vi "Main.vi"() -> ()   [LabVIEW 2013]
uses:
  <vilib>/Platform/TimedLoop/XDataNode/timing_clust.ctl
  <vilib>/Platform/TimedLoop/XDataNode/nitl_modes.ctl
  <vilib>/Platform/TimedLoop/XDataNode/wakeup.ctl
  <vilib>/Utility/file.llb/Write To Spreadsheet File (DBL).vi
  <vilib>/platform/TimedLoop/XDataNode/XDataNode.xnode
  <vilib>/Platform/TimedLoop/XDataNode/XDNodeRunTimeDep.lvlib
panel:
  out "X-axis acceleration [g]":dbl(knob) scale=-2.0..2.0
  out "Acquired data":cluster{dbl[], dbl[]}(graph)
  in  "[ESC]":bool
  in  "logfile base name":string="logfile"
  out "logfile name":path
  out "USB flash drive info":string
  out "folder names":string[](array[string])
  out "filenames":string[](array[string])
  # "USB Flash Drive demo"
  # "1. Insert USB flash drive\n2. Enter logfile base name\n3. Run the VI\n4. Move NI myRIO to see onboard\n    accelerometer activity\n5. Stop the VI to save\n    acquired acceleration data to\n    logfile on USB flash drive"
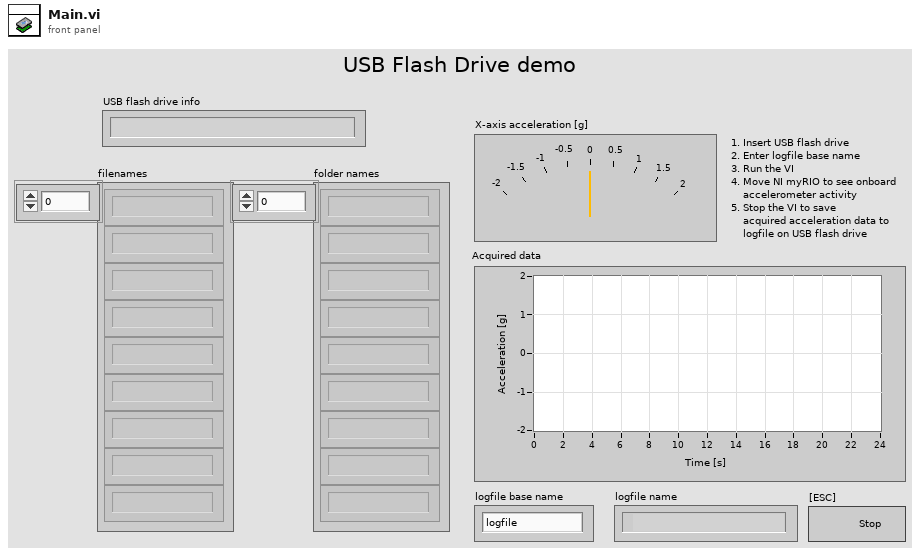
[diagram p1: front panel]
types:
  T1 = typedef "XDNodeRunTimeDep.lvlib/timing_clust.ctl" = cluster{"Expected End [f-1]":u64, "Actual End [f-1]":u64, "Finished Late? [f-1]":bool, "Expected End [i-1]":u64, "Actual End [i-1]":u64, "Finished Late? [i-1]":bool, "Expected Start [i]":u64, "Actual Start [i]":u64, "Expected Start [f]":u64, "Actual Start [f]":u64, "Source Name":string, "Structure Name":string, "Period":i64, "Deadline":i64, "Offset":i64, "Start":i64, "Priority":i32, "Timeout":i32, "Mode":T2, "Wakeup Reason":T3, "Error":errorcluster, "Source Type":string, "Secondary Source Type":string, "Global End Time":u64, "Global Start Time":u64, "Frame Duration":u64, "Iteration Duration":u64, "Assigned CPU":i32, "I/O Scan Engine Mode":u32}
  T2 = typedef "XDNodeRunTimeDep.lvlib/nitl_modes.ctl" = enum32{"No Change", "Process missed periods, maintain original phase", "Discard missed periods, maintain original phase", "Process missed periods, ignore original phase", "Discard missed periods, ignore original phase"}
  T3 = typedef "XDNodeRunTimeDep.lvlib/wakeup.ctl" = enum32{"Normal", "Aborted", "Asynchronous wakeup", "Timing source error", "Timed loop error", "Timeout"}
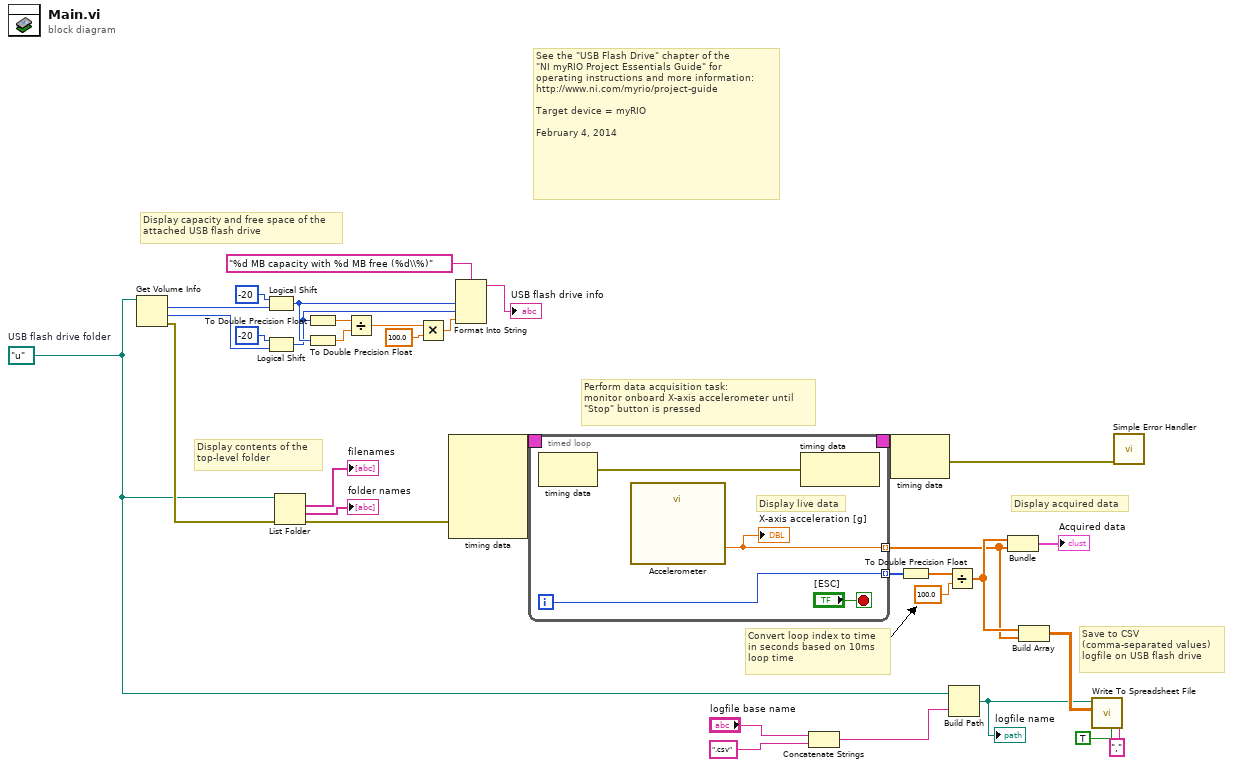
[diagram p0: block diagram]
diagram:
  w1 = path "u:/"  # USB flash drive folder
  # "See the \"USB Flash Drive\" chapter of the\n\"NI myRIO Project Essentials Guide\" for\noperating instructions and more information: \nhttp://www.ni.com/myrio/project-guide\n\nTarget device = myRIO\n\nFebruary 4, 2014"
  # "Convert loop index to time\nin seconds based on 10ms\nloop time"
  # "Display acquired data"
  # "Save to CSV\n(comma-separated values)\nlogfile on USB flash drive"
  # "Perform data acquisition task:\nmonitor onboard X-axis accelerometer until\n\"Stop\" button is pressed"
  # "Display contents of the \ntop-level folder"
  # "Display capacity and free space of the\nattached USB flash drive"
  n1 = Get Volume Info(11:w1) -> (0:w19:errorcluster, 1:w32:i64, 2:w28:i64)  [unwired: 1 in, 3 out]
  n2 = Logical Shift(y=i16 -20, x=w28) -> (x << y=w23:i64)
  n3 = Logical Shift(y=i16 -20, x=w32) -> (x << y=w21:i64)
  n4 = List Folder(path=w1, error in=w19) -> (filenames=→"filenames":string[], folder names=→"folder names":string[], error out=w13:errorcluster)  [unwired: 2 in, 1 out]
  n5 = To Double Precision Float(number=w21) -> (double precision float=w20:dbl)
  n6 = To Double Precision Float(number=w23) -> (double precision float=w22:dbl)
  n7 = Divide(x=w20, y=w22) -> (x/y=w26:dbl)
  n8 = Multiply(x=w26, y=100.0) -> (x*y=w24:dbl)
  n9 = node-c288(w13) -> (w15:T1)  [unwired: 4 in]
  n10 = Format Into String "Format Into String"(format string="%d MB capacity with %d MB free (%d\\%)", w23, w21, w24) -> (resulting string=→"USB flash drive info":string)  [unwired: 2 in, 1 out]
  n11 = timed-loop {
    timing: w15 -> [_]
    timing-out: [_] -> w14
    tunnel: [w35] -> w7 mode=indexing
    tunnel: [w36] -> w12 mode=indexing
    i -> [w36]
    stop <- "[ESC]" stop-if-true
    # "Display live data"
    n12 = node-c288() -> (w37:errorcluster)  [unwired: 1 in]
    n13 = call "Accelerometer"() -> ("X-Axis"=w35:dbl)  [unwired: 26 in, 1 out]
    "X-axis acceleration [g]" <- w35
    n14 = node-c288(w37) -> ()  [unwired: 1 out]
  }
  n15 = Concatenate Strings "Concatenate Strings"("logfile base name", ".csv" ("string")) -> (w16:string)
  n16 = node-c288(w14) -> (w3:errorcluster)
  n17 = To Double Precision Float(number=w12) -> (double precision float=w10:dbl[])
  n18 = Divide(x=w10, y=100.0) -> (x/y=w8:dbl[])
  n19 = Build Path(base path=w1, name or relative path=w16) -> (appended path=w5:path)
  "logfile name" <- w5
  n20 = Bundle "Bundle"(w8, w7) -> (→"Acquired data":cluster{dbl[], dbl[]})  [unwired: 1 in]
  n21 = Build Array "Build Array"(w8, w7) -> (w6:dbl[][])
  n22 = call-poly <vilib>:"Write To Spreadsheet File.vi"("delimiter (\\t)"="," ("delimiter (\\t)"), "transpose? (no:F)"=TRUE, "2D data"=w6, "file path (dialog if empty)"=w5) -> ()  [unwired: 4 in, 1 out]
  n23 = call <vilib>:"Simple Error Handler.vi"("error in (no error)"=w3) -> ()  [unwired: 4 in, 5 out]
